vi "CH_LM App Statistics PtByPt.vi"(2 "initialize":bool, 3 "x":dbl format="%0.2f") -> (0 "standard deviation":dbl format="%0.2f", 1 "mean":dbl format="%0.2f")   [LabVIEW 2012, in "CH_LM App.lvlib"]
doc: "This VI is used to calculate mean and standard deviation of incoming x values."
uses:
  CH_LM App.lvlib
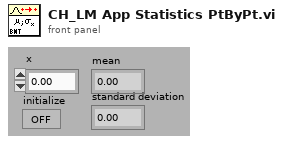
[diagram p1: front panel]
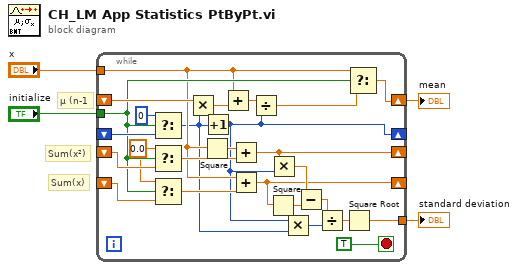
[diagram p0: block diagram]
diagram:
  # "Sum(x²)"
  # "Sum(x)"
  # "µ (n-1"
  n1 = while {
    shift-right: [w30] -> w2
    shift-left: _ -> [w26]
    tunnel: "initialize" -> [w18]
    tunnel: "x" -> [w11]
    shift-right: [w5] -> _
    shift-left: _ -> [w27]
    shift-right: [w9] -> _
    shift-left: _ -> [w22]
    shift-right: [w8] -> _
    shift-left: _ -> [w20]
    tunnel: [w14] -> w1
    stop <- TRUE stop-if-true
    w17 = 0.0 ("t")
    n2 = Select(t=u64 0, s=w18, f=w27) -> (s? t:f=w6:u64)
    n3 = Select(t=w17, s=w18, f=w22) -> (s? t:f=w21:dbl)
    n4 = Select(t=w17, s=w18, f=w20) -> (s? t:f=w19:dbl)
    n5 = Multiply(x=w26, y=w6) -> (x*y=w25:dbl)
    n6 = Square(x=w11) -> (x^2=w10:dbl)
    n7 = Increment(x=w6) -> (x+1=w5:u64)
    n8 = Add(x=w11, y=w25) -> (x+y=w24:dbl)
    n9 = Add(x=w10, y=w21) -> (x+y=w9:dbl)
    n10 = Add(x=w11, y=w19) -> (x+y=w8:dbl)
    n11 = Divide(x=w24, y=w5) -> (x/y=w23:dbl)
    n12 = Square(x=w8) -> (x^2=w12:dbl)
    n13 = Multiply(x=w9, y=w5) -> (x*y=w13:dbl)
    n14 = Multiply(x=w5, y=w6) -> (x*y=w16:u64)
    n15 = Subtract(x=w13, y=w12) -> (x-y=w7:dbl)
    n16 = Divide(x=w7, y=w16) -> (x/y=w15:dbl)
    n17 = Square Root(x=w15) -> (sqrt(x)=w14:dbl)
    n18 = Select(t=w11, s=w18, f=w23) -> (s? t:f=w30:dbl)
  }
  "standard deviation" <- w1
  "mean" <- w2
